vi "Build Initial Conditions Cluster.vi"(5 "User VI Path":path, 6 "Owner Filename":string, 7 "Project Refs":refnum<vi>[](array[refnum]), 8 "Virtual Folder Search Results":T2, 9 "User VI Owner Status":T3, 10 "Multiple lvproj open?":bool, 11 "Exactly one lvproj open?":bool) -> (3 "Input Conditions":T1)   [LabVIEW 2022 SP3]
doc: "<add documentation here>"
uses:
  Owner Status (enum).ctl
  DFS Output (cluster).ctl
  Input Conditions (cluster).ctl
panel:
  # "Development\nControls or indicators that are useful for development or testing, but which are not outputs of the VI."
  # "Input\nInputs to the VI"
  # "Output\nOutputs of the VI"
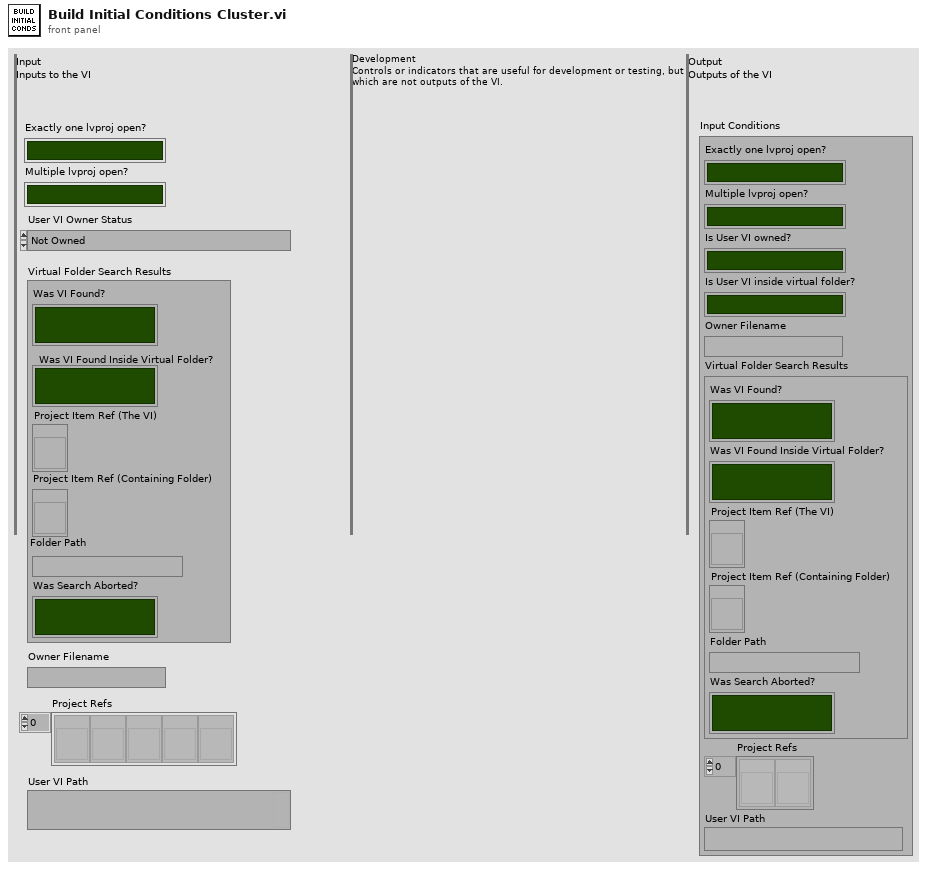
[diagram p1: front panel]
types:
  T1 = typedef "Input Conditions (cluster).ctl" = cluster{"Exactly one lvproj open?":bool, "Multiple lvproj open?":bool, "Is User VI owned?":bool, "Is User VI inside virtual folder?":bool, "Owner Filename":string, "Virtual Folder Search Results":T2, "Project Refs":refnum<vi>[], "User VI Path":path}
  T2 = typedef "DFS Output (cluster).ctl" = cluster{"Was VI Found?":bool, "Was VI Found Inside Virtual Folder?":bool, "Project Item Ref (The VI)":refnum<vi>, "Project Item Ref (Containing Folder)":refnum<vi>, "Folder Path":string, "Was Search Aborted?":bool}
  T3 = typedef "Owner Status (enum).ctl" = enum16{"Not Owned", "Owned by Library (lvlib)", "Owned by Class (lvclass)"}
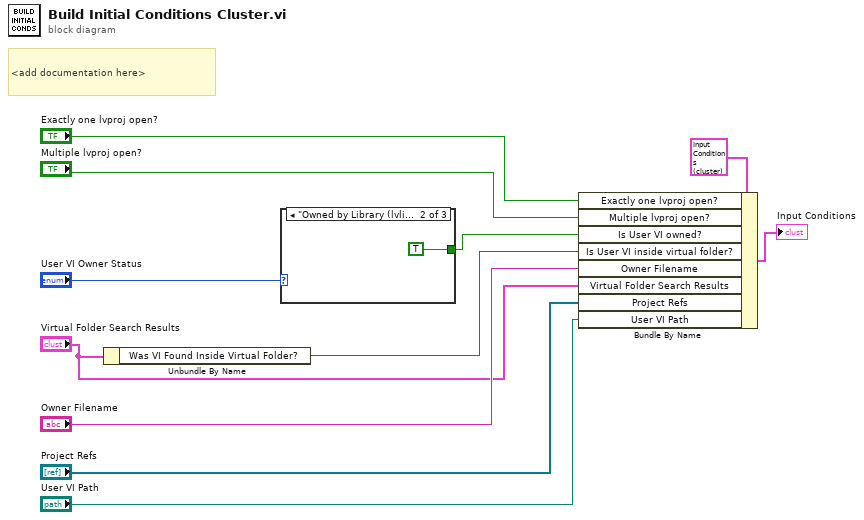
[diagram p0: block diagram]
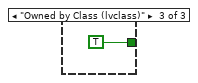
[diagram p3: hidden frame]
diagram:
  # "<add documentation here>"
  n1 = Unbundle By Name("Virtual Folder Search Results") -> ("Was VI Found Inside Virtual Folder?"=w9:bool)
  n2 = case shown="\"Owned by Library (lvlib)\"" "User VI Owner Status" {
    tunnel: [_ TRUE TRUE] -> w7
    frame "Not Owned" {
    }
    frame "Owned by Library (lvlib)" {
    }
    frame "Owned by Class (lvclass)" {
    }
  }
  n3 = Bundle By Name(cluster=T1 {"Exactly one lvproj open?"=FALSE, "Multiple lvproj open?"=FALSE, "Is User VI owned?"=FALSE, "Is User VI inside virtual folder?"=FALSE, "Owner Filename"="", "Virtual Folder Search Results"={"Was VI Found?"=FALSE, "Was VI Found Inside Virtual Folder?"=FALSE, "Project Item Ref (The VI)"=refnum, "Project Item Ref (Containing Folder)"=refnum, "Folder Path"="", "Was Search Aborted?"=FALSE}, "Project Refs"=[], "User VI Path"=path ""} ("Input Conditions"), "Exactly one lvproj open?"="Exactly one lvproj open?", "Multiple lvproj open?"="Multiple lvproj open?", "Is User VI owned?"=w7, "Is User VI inside virtual folder?"=w9, "Owner Filename"="Owner Filename", "Virtual Folder Search Results"="Virtual Folder Search Results", "Project Refs"="Project Refs", "User VI Path"="User VI Path") -> (→"Input Conditions":T1)
